vi "求最大值.vi"() -> ()   [LabVIEW 2009]
panel:
  out "求100个随机数的最大值":dbl
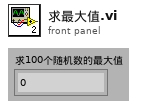
[diagram p1: front panel]
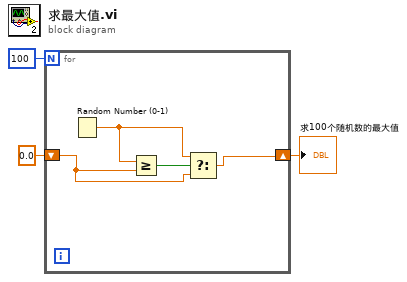
[diagram p0: block diagram]
diagram:
  n1 = for {
    N: 100 -> [_]
    shift-right: [w5] -> w1
    shift-left: 0.0 ("number: 0 to 1") -> [w4]
    n2 = Random Number (0-1)() -> (number: 0 to 1=w6:dbl)
    n3 = Greater Or Equal?(x=w6, y=w4) -> (x >= y?=w7:bool)
    n4 = Select(t=w6, s=w7, f=w4) -> (s? t:f=w5:dbl)
  }
  "求100个随机数的最大值" <- w1
